vi "Drive Reef Align.vi"(4 "Auto Data":T2, 6 "Operation":T3=enum."Reef Align", 7 "Description":string, 8 "Command Info In":T4, 9 "Angle Align":bool, 10 "Left Side?":bool, 11 "Robot Velocities":T1) -> (0 "Command Info Out":T4)   [LabVIEW 2023]
doc: "This VI notifies the subsystem to the new setpoint."
uses:
  <vilib>/Rock Robotics/WPI/Framework/Command Status Info.ctl
  <vilib>/Rock Robotics/WPI/Framework/Completion Status.ctl
  <vilib>/Rock Robotics/WPI/Framework/Completion Notifier.ctl
  swerve/Type Definitions/Data/Robot Velocities.ctl
  Implementation/Drive Operations.ctl
  Implementation/Drive Setpoints.ctl
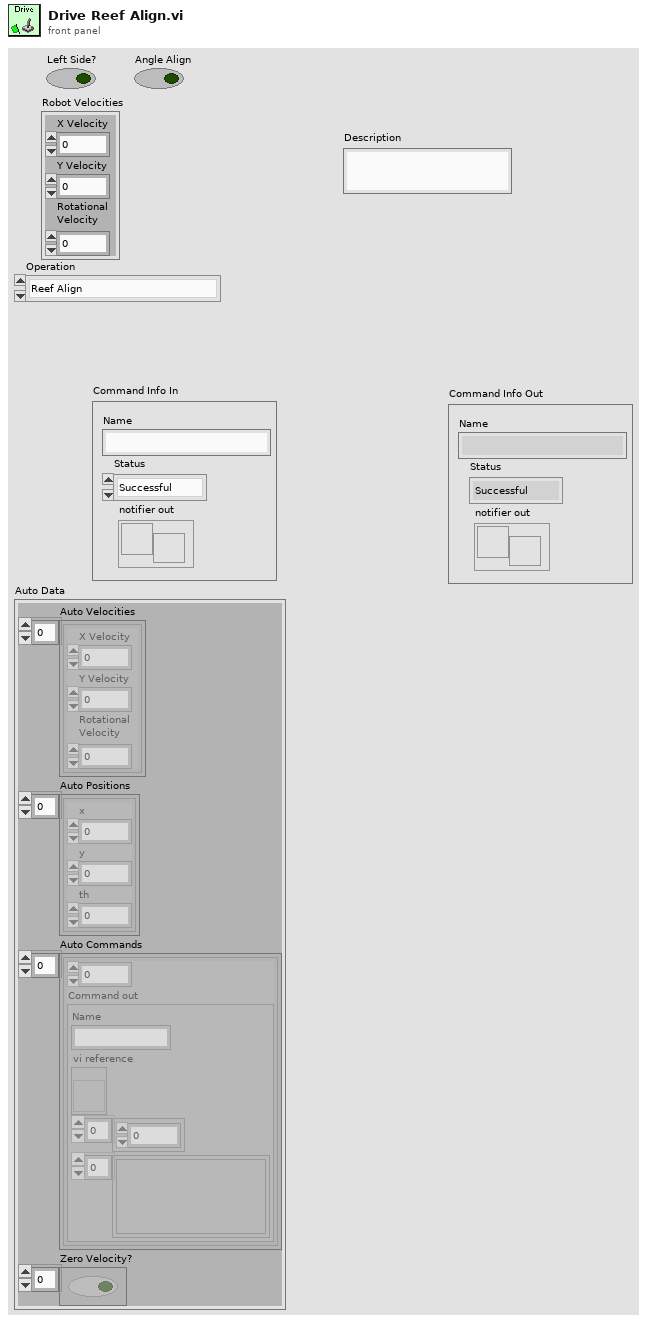
[diagram p1: front panel]
types:
  T1 = typedef "Robot Velocities.ctl" = cluster{"X Velocity":dbl, "Y Velocity":dbl, "Rotational \nVelocity":dbl}
  T2 = cluster{"Auto Velocities":T1[], "Auto Positions":cluster{"x":dbl, "y":dbl, "th":dbl}[], "Auto Commands":cluster{dbl, "Command out":cluster{"Name":string, "vi reference":refnum<vi>, i32[], variant[]}}[], "Zero Velocity?":bool[]}
  T3 = typedef "Drive Operations.ctl" = enum16{"Reserve", "Read Current", "Immediate", "Calibrate", "Reef Align", "Auto"}
  T4 = typedef "Command Status Info.ctl" = cluster{"Name":string, "Status":T5, "notifier out":T6}
  T5 = typedef "Completion Status.ctl" = enum16{"Successful", "Aborted", "Incomplete"}
  T6 = typedef "Completion Notifier.ctl" = refnum<notifier>
  T7 = typedef "Drive Setpoints.ctl" = cluster{"Operation":T3, "Robot Velocities":T1, "Auto Data":cluster{"Auto Velocities":T1[], "Auto Positions":cluster{"x":dbl, "y":dbl, "th":dbl}[], "Auto Commands":cluster{dbl, "Command out":cluster{"Name":string, "vi reference":refnum<vi>, i32[], variant[]}}[], "Zero Velocity?":bool[]}, "Left side":bool, "Angle Align":bool, "Tag ID":i32}
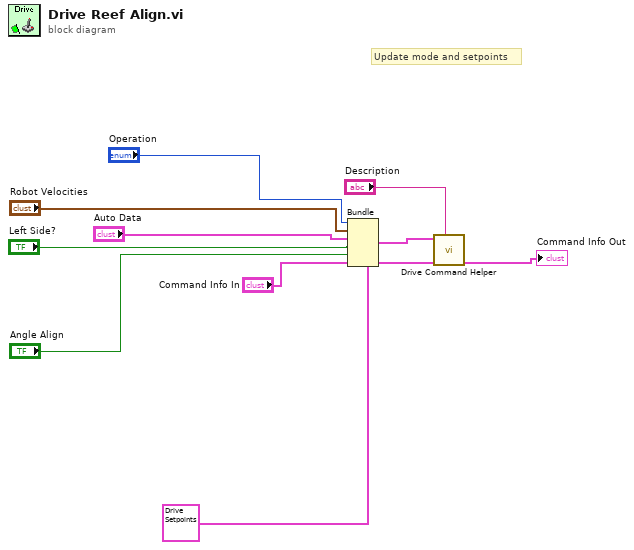
[diagram p0: block diagram]
diagram:
  # "Update mode and setpoints"
  n1 = Bundle(cluster=T7 {"Operation"=enum."Reef Align", "Robot Velocities"={"X Velocity"=0.0, "Y Velocity"=0.0, "Rotational \nVelocity"=0.0}, "Auto Data"={"Auto Velocities"=[], "Auto Positions"=[], "Auto Commands"=[], "Zero Velocity?"=[]}, "Left side"=FALSE, "Angle Align"=FALSE, "Tag ID"=0} ("SubSystem Data"), "Operation"="Operation", "Robot Velocities"="Robot Velocities", "Auto Data"="Auto Data", "Left side"="Left Side?", "Angle Align"="Angle Align") -> (w5:T7)  [unwired: 1 in]
  n2 = call "Drive Command Helper.vi"("Description"="Description", "Command Info In"="Command Info In", "SubSystem Data"=w5) -> ("Command Info Out"=→"Command Info Out":T4)  [unwired: 6 in, 2 out]
